vi "HAPS_MCU_Preamp_CMD.vi"(5 "set_Preamp":T3={"ch"=0, "chain_id"=0, "group"=3, "array_id"=0, "ele_phase"=0, "ele_gain"=0, "com_gain"=0, "pd_range"=0}, 7 "HAPS_MCU_Preamp_Func.":T2(ring), 8 "error in":errorcluster, 11 "Function":T1={"Tx/Rx"=enum."Rx", "Enable?"=enum."On", "Source"=enum."MCU"}) -> (0 "error out":errorcluster, 3 "Data":string)   [LabVIEW 2023, in "HAPS.lvlib"]
uses:
  HAPS.lvlib
  set_Preamp.ctl
  MCU_Function.ctl
panel:
  out "Time(ms)":dbl
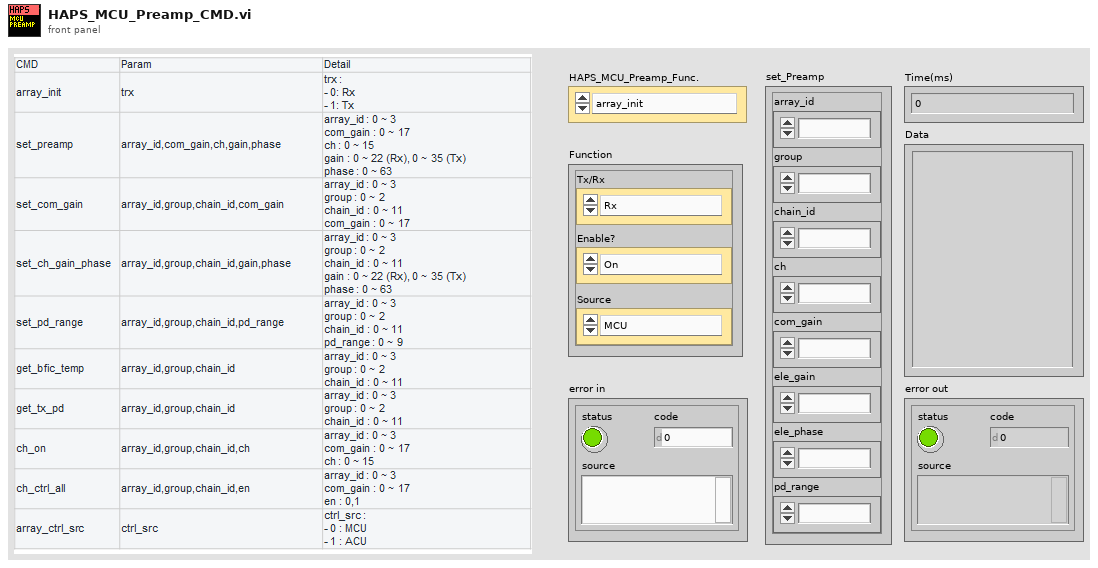
[diagram p1: front panel]
types:
  T1 = typedef "HAPS.lvlib/MCU_Function.ctl" = cluster{"Tx/Rx":enum16{"Rx", "Tx"}, "Enable?":enum16{"OFF", "On"}, "Source":enum16{"MCU", "ACU"}}
  T2 = enum16{"array_init", "set_preamp", "set_com_gain", "set_ch_gain_phase", "set_pd_range", "get_bfic_temp", "get_tx_pd", "ch_on", "ch_ctrl_all", "array_ctrl_src"}
  T3 = typedef "HAPS.lvlib/set_Preamp.ctl" = cluster{"ch":i32, "chain_id":i32, "group":i32, "array_id":i32, "ele_phase":i32, "ele_gain":i32, "com_gain":i32, "pd_range":i32}
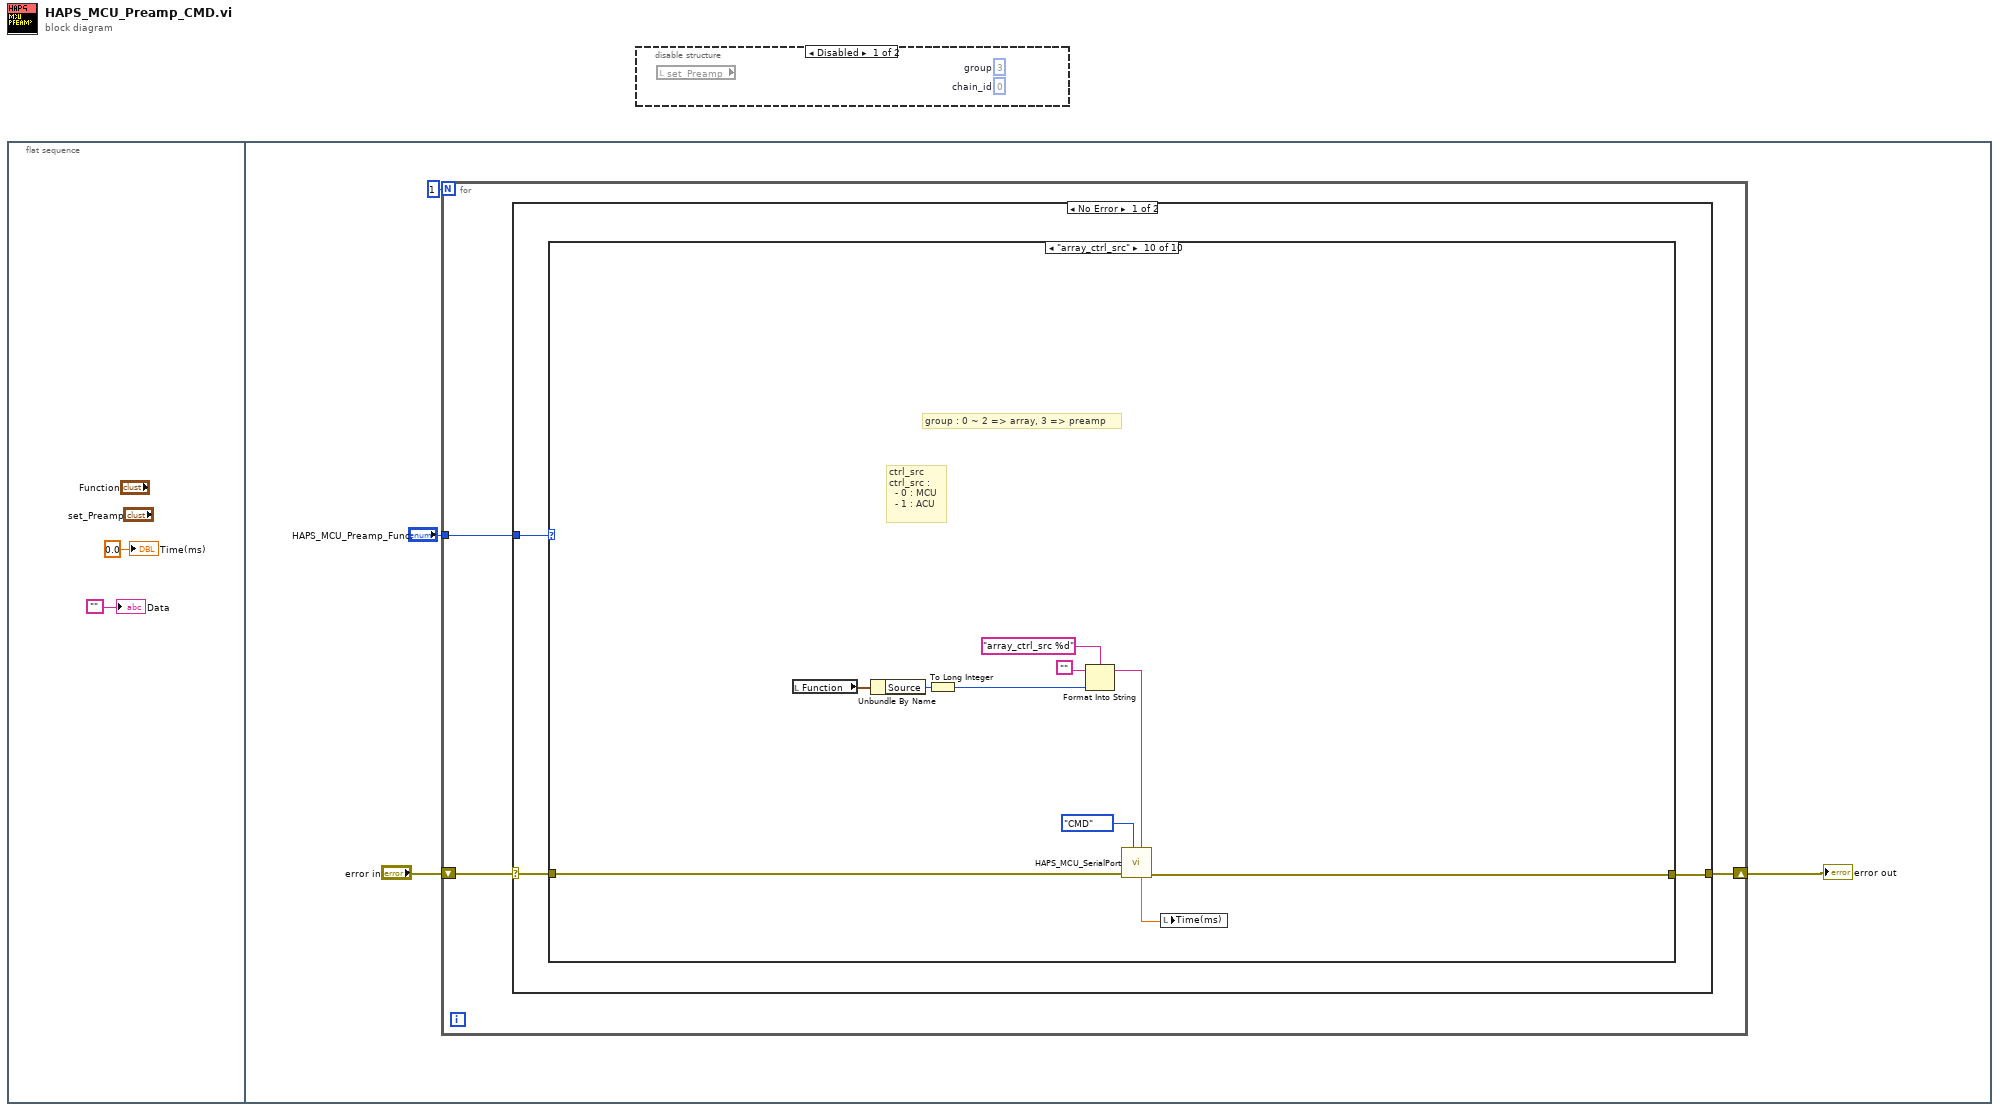
[diagram p0: block diagram]
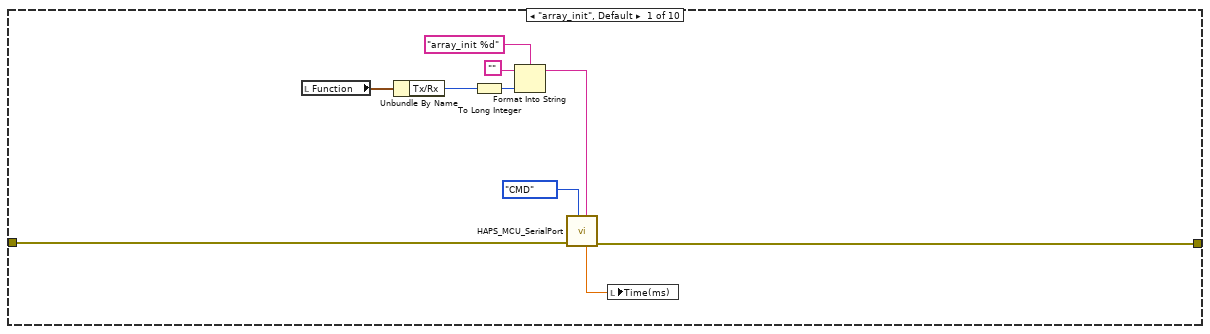
[diagram p3: hidden frame]
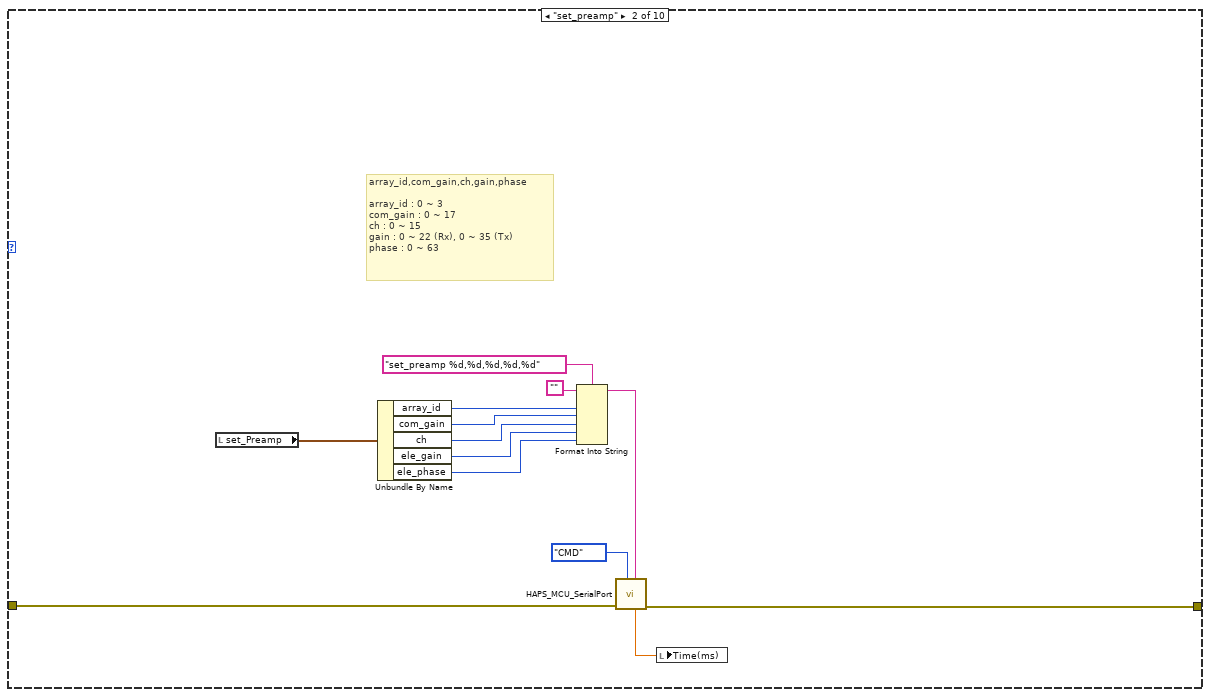
[diagram p4: hidden frame]
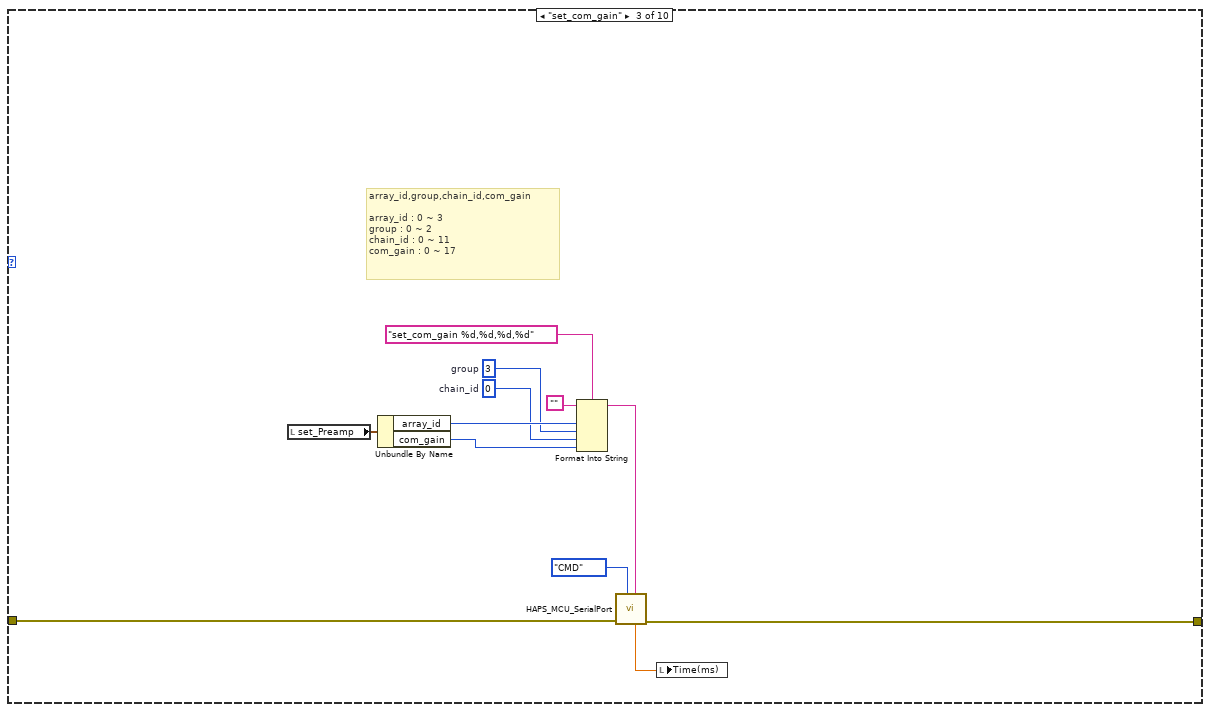
[diagram p5: hidden frame]
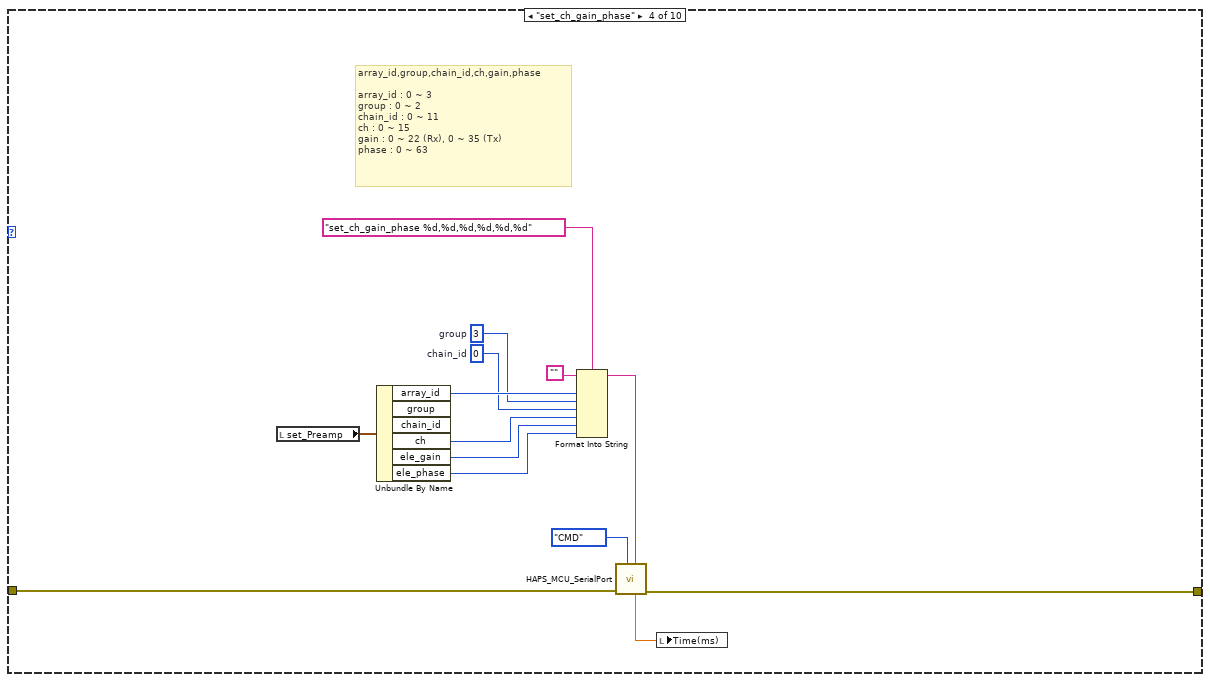
[diagram p6: hidden frame]
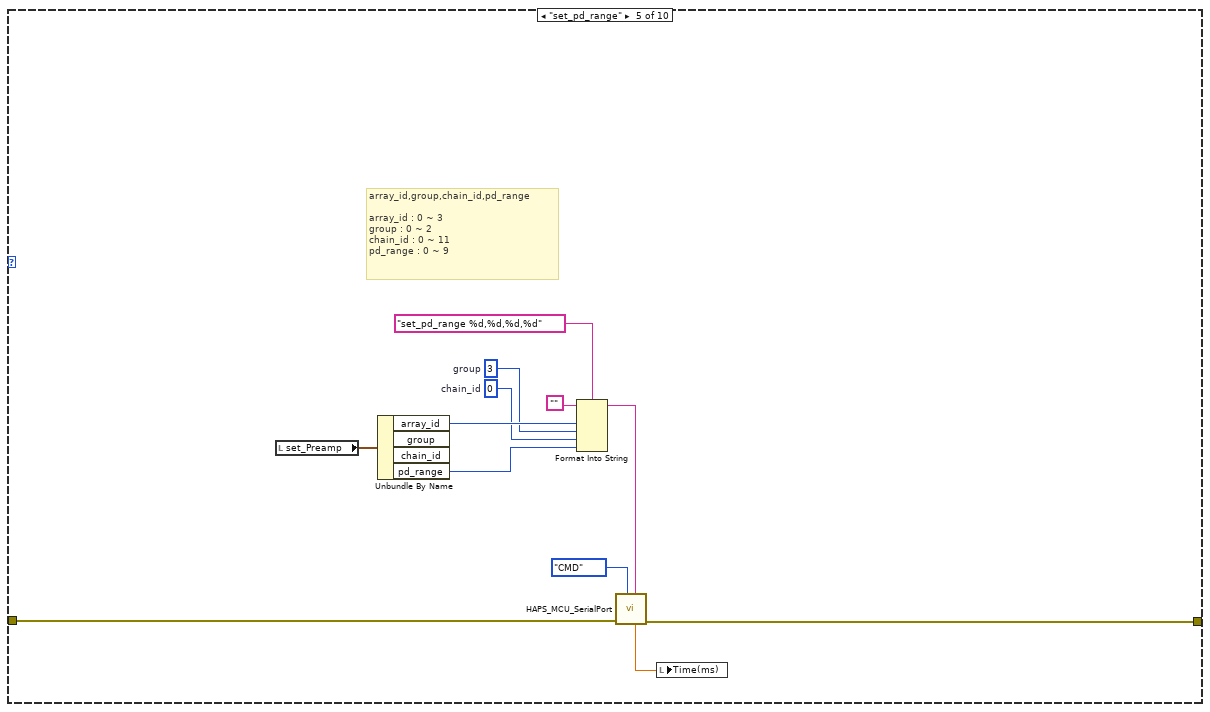
[diagram p7: hidden frame]
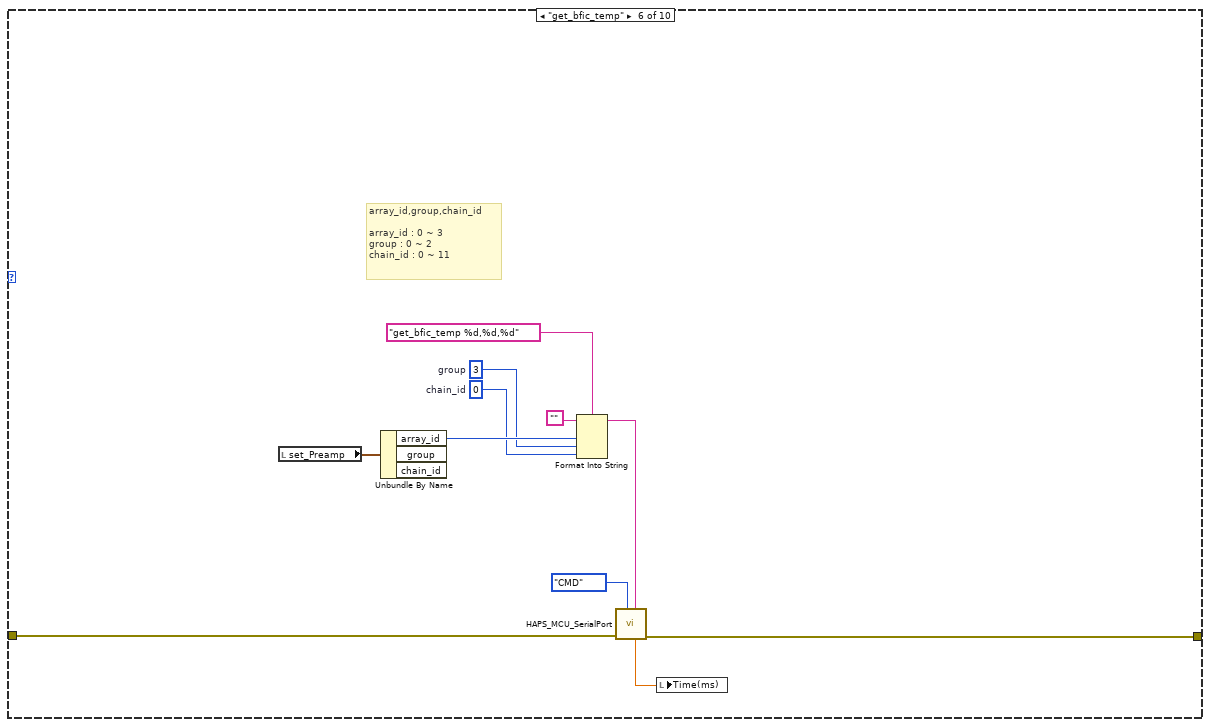
[diagram p8: hidden frame]
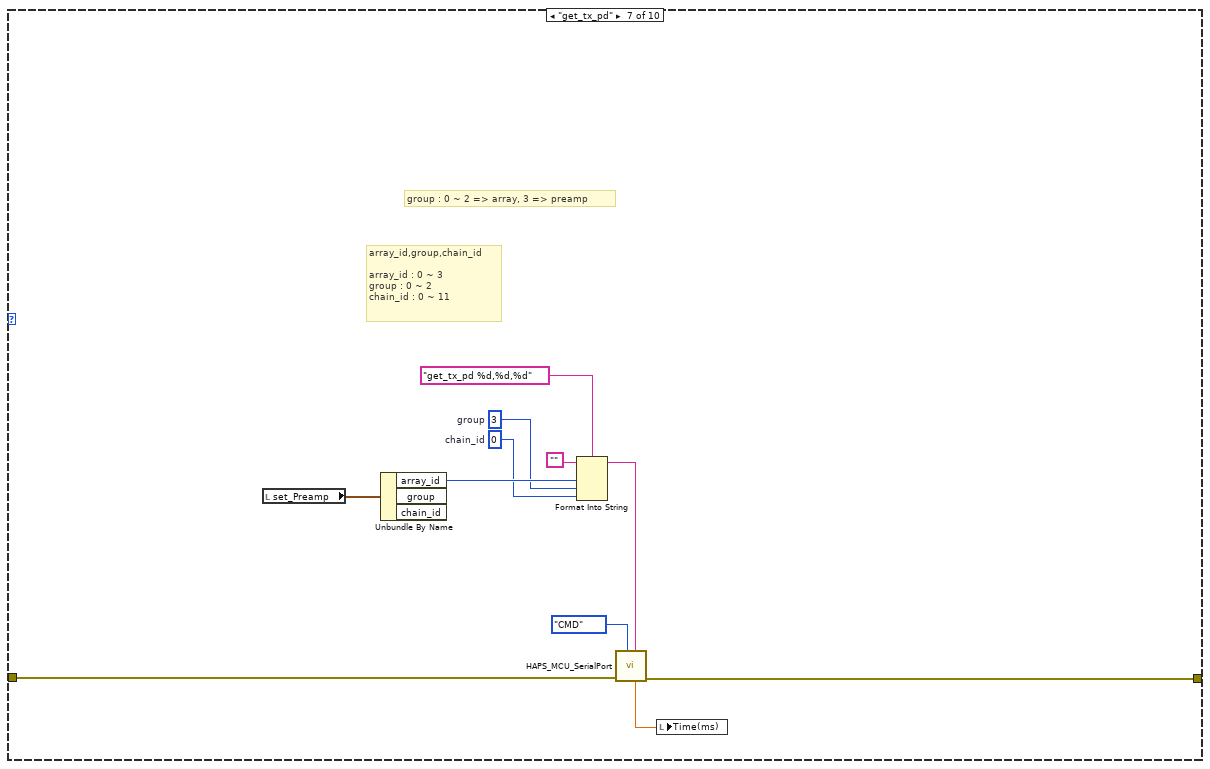
[diagram p9: hidden frame]
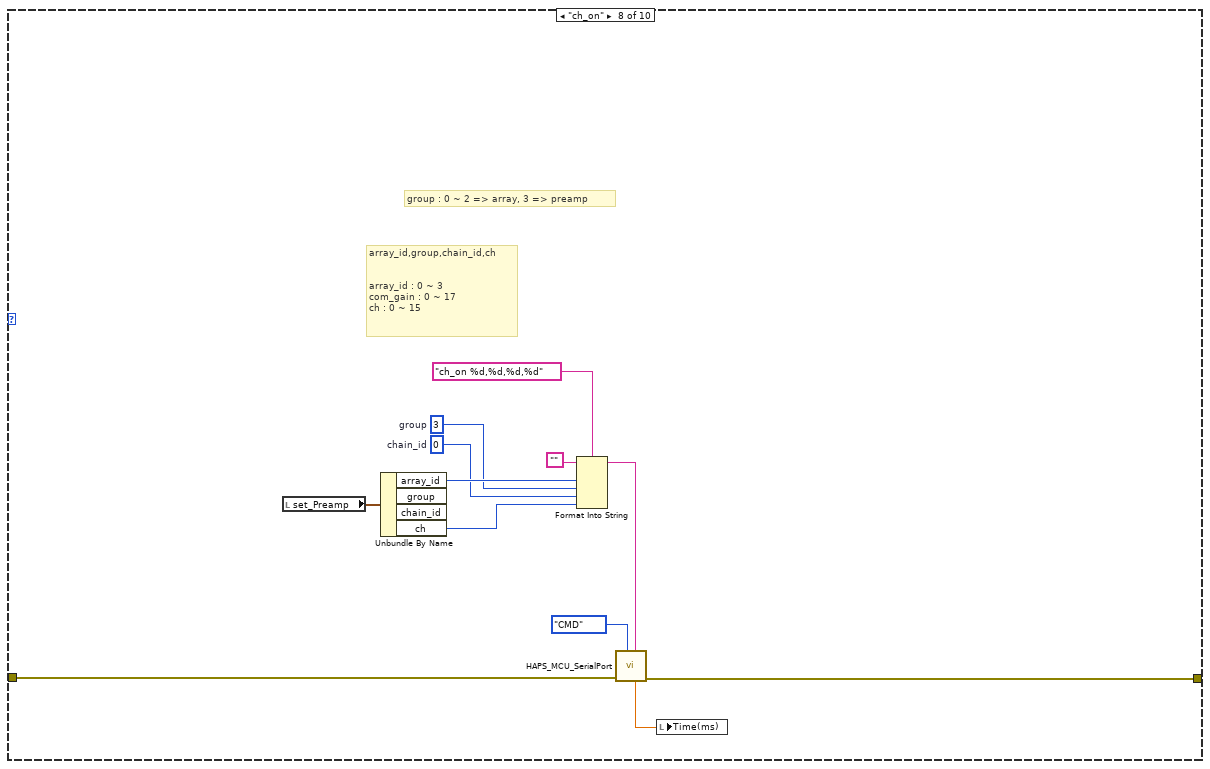
[diagram p10: hidden frame]
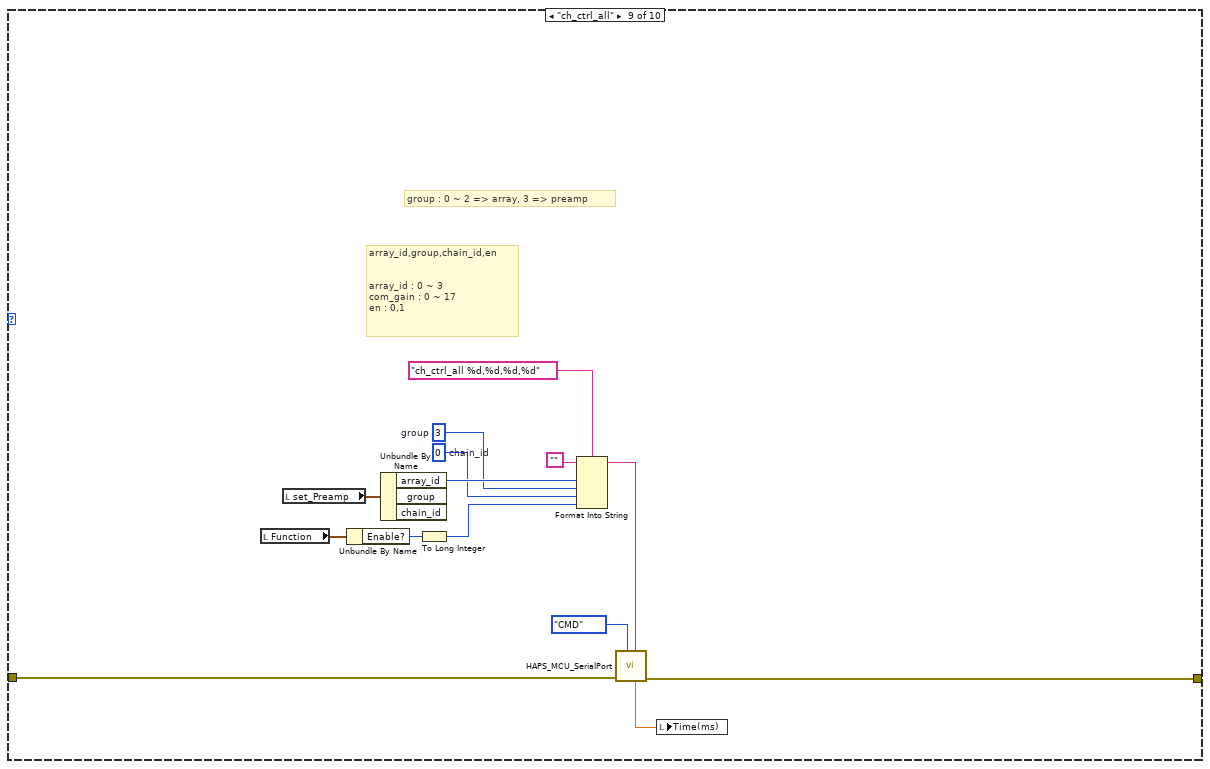
[diagram p11: hidden frame]
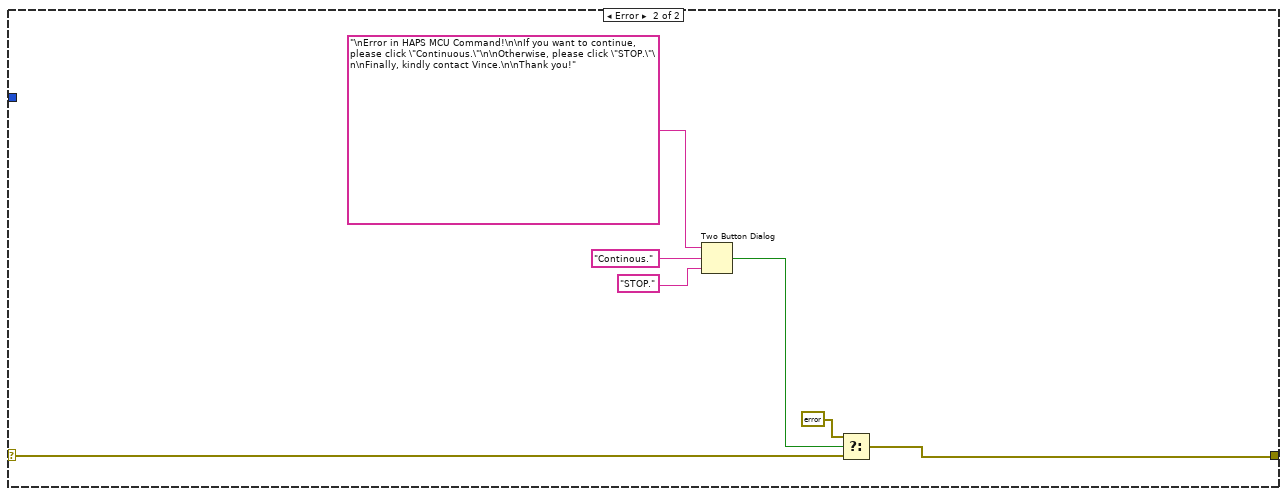
[diagram p12: hidden frame]
diagram:
  n1 = flat-sequence {
    frame #0 {
      "Time(ms)" <- 0.0 ("Time(ms)")
      "Data" <- ""
    }
    frame #1 {
      n2 = for {
        N: 1 -> [_]
        tunnel: "HAPS_MCU_Preamp_Func." -> [w7]
        shift-right: [w9] -> w3
        shift-left: "error in" -> [w8]
        n3 = case shown="No Error" w8 {
          selector: w8 -> [w12 w134]
          tunnel: [w10 w132] -> w9
          tunnel: w7 -> [w11 _]
          frame No Error {
            n4 = case shown="\"array_ctrl_src\"" w11 {
              tunnel: w12 -> [w22 w35 w47 w61 w73 w84 w95 w107 w121 w131]
              tunnel: [w21 w34 w46 w60 w72 w83 w94 w106 w120 w130] -> w10
              frame "array_init", Default {
                n5 = local read "Function"() -> (w16:T1)
                n6 = Unbundle By Name(w16) -> ("Tx/Rx"=w13:enum16{"Rx", "Tx"})
                n7 = To Long Integer(number=w13) -> (32bit integer=w15:i32)
                n8 = Format Into String(format string="array_init %d" ("Command"), initial string="", w15) -> (resulting string=w14:string)  [unwired: 1 in, 1 out]
                n9 = call "HAPS_MCU_SerialPort.vi"("Command"=w14, "HAPS_SerialPort_Func"=enum16{"Init", "Close", "CMD"}."CMD" ("HAPS_SerialPort"), "error in"=w22) -> ("error out"=w21:errorcluster, "Time(ms)"=w20:dbl)  [unwired: 6 in, 1 out]
                n10 = local write "Time(ms)"(w20) -> ()
              }
              frame "set_preamp" {
                # "array_id,com_gain,ch,gain,phase\n\narray_id : 0 ~ 3\ncom_gain : 0 ~ 17\nch : 0 ~ 15\ngain : 0 ~ 22 (Rx), 0 ~ 35 (Tx)\nphase : 0 ~ 63"
                n11 = local read "set_Preamp"() -> (w23:T3)
                n12 = Unbundle By Name(w23) -> ("array_id"=w28:i32, "com_gain"=w27:i32, "ch"=w26:i32, "ele_gain"=w25:i32, "ele_phase"=w24:i32)
                n13 = Format Into String(format string="set_preamp %d,%d,%d,%d,%d" ("Command"), initial string="", w28, w27, w26, w25, w24) -> (resulting string=w29:string)  [unwired: 1 in, 1 out]
                n14 = call "HAPS_MCU_SerialPort.vi"("Command"=w29, "HAPS_SerialPort_Func"=enum16{"Init", "Close", "CMD"}."CMD" ("HAPS_SerialPort"), "error in"=w35) -> ("error out"=w34:errorcluster, "Time(ms)"=w33:dbl)  [unwired: 6 in, 1 out]
                n15 = local write "Time(ms)"(w33) -> ()
              }
              frame "set_com_gain" {
                w37 = 0  # chain_id
                w38 = 3  # group
                # "array_id,group,chain_id,com_gain\n\narray_id : 0 ~ 3\ngroup : 0 ~ 2\nchain_id : 0 ~ 11\ncom_gain : 0 ~ 17"
                n16 = local read "set_Preamp"() -> (w39:T3)
                n17 = Unbundle By Name(w39) -> ("array_id"=w40:i32, "com_gain"=w36:i32)
                n18 = Format Into String(format string="set_com_gain %d,%d,%d,%d" ("Command"), initial string="", w40, w38, w37, w36) -> (resulting string=w41:string)  [unwired: 1 in, 1 out]
                n19 = call "HAPS_MCU_SerialPort.vi"("Command"=w41, "HAPS_SerialPort_Func"=enum16{"Init", "Close", "CMD"}."CMD" ("HAPS_SerialPort"), "error in"=w47) -> ("error out"=w46:errorcluster, "Time(ms)"=w45:dbl)  [unwired: 6 in, 1 out]
                n20 = local write "Time(ms)"(w45) -> ()
              }
              frame "set_ch_gain_phase" {
                w48 = 0  # chain_id
                w49 = 3  # group
                # "array_id,group,chain_id,ch,gain,phase\n\narray_id : 0 ~ 3\ngroup : 0 ~ 2\nchain_id : 0 ~ 11\nch : 0 ~ 15\ngain : 0 ~ 22 (Rx), 0 ~ 35 (Tx)\nphase : 0 ~ 63"
                n21 = local read "set_Preamp"() -> (w52:T3)
                n22 = Unbundle By Name(w52) -> ("array_id"=w54:i32, "ch"=w53:i32, "ele_gain"=w51:i32, "ele_phase"=w50:i32)  [unwired: 2 out]
                n23 = Format Into String(format string="set_ch_gain_phase %d,%d,%d,%d,%d,%d" ("Command"), initial string="", w54, w49, w48, w53, w51, w50) -> (resulting string=w55:string)  [unwired: 1 in, 1 out]
                n24 = call "HAPS_MCU_SerialPort.vi"("Command"=w55, "HAPS_SerialPort_Func"=enum16{"Init", "Close", "CMD"}."CMD" ("HAPS_SerialPort"), "error in"=w61) -> ("error out"=w60:errorcluster, "Time(ms)"=w59:dbl)  [unwired: 6 in, 1 out]
                n25 = local write "Time(ms)"(w59) -> ()
              }
              frame "set_pd_range" {
                w63 = 0  # chain_id
                w62 = 3  # group
                # "array_id,group,chain_id,pd_range\n\narray_id : 0 ~ 3\ngroup : 0 ~ 2\nchain_id : 0 ~ 11\npd_range : 0 ~ 9"
                n26 = local read "set_Preamp"() -> (w64:T3)
                n27 = Unbundle By Name(w64) -> ("array_id"=w66:i32, "pd_range"=w65:i32)  [unwired: 2 out]
                n28 = Format Into String(format string="set_pd_range %d,%d,%d,%d" ("Command"), initial string="", w66, w62, w63, w65) -> (resulting string=w67:string)  [unwired: 1 in, 1 out]
                n29 = call "HAPS_MCU_SerialPort.vi"("Command"=w67, "HAPS_SerialPort_Func"=enum16{"Init", "Close", "CMD"}."CMD" ("HAPS_SerialPort"), "error in"=w73) -> ("error out"=w72:errorcluster, "Time(ms)"=w71:dbl)  [unwired: 6 in, 1 out]
                n30 = local write "Time(ms)"(w71) -> ()
              }
              frame "get_bfic_temp" {
                w75 = 0  # chain_id
                w74 = 3  # group
                # "array_id,group,chain_id\n\narray_id : 0 ~ 3\ngroup : 0 ~ 2\nchain_id : 0 ~ 11"
                n31 = local read "set_Preamp"() -> (w76:T3)
                n32 = Unbundle By Name(w76) -> ("array_id"=w77:i32)  [unwired: 2 out]
                n33 = Format Into String(format string="get_bfic_temp %d,%d,%d" ("Command"), initial string="", w77, w74, w75) -> (resulting string=w78:string)  [unwired: 1 in, 1 out]
                n34 = call "HAPS_MCU_SerialPort.vi"("Command"=w78, "HAPS_SerialPort_Func"=enum16{"Init", "Close", "CMD"}."CMD" ("HAPS_SerialPort"), "error in"=w84) -> ("error out"=w83:errorcluster, "Time(ms)"=w82:dbl)  [unwired: 6 in, 1 out]
                n35 = local write "Time(ms)"(w82) -> ()
              }
              frame "get_tx_pd" {
                w86 = 0  # chain_id
                w85 = 3  # group
                # "group : 0 ~ 2 => array, 3 => preamp"
                # "array_id,group,chain_id\n\narray_id : 0 ~ 3\ngroup : 0 ~ 2\nchain_id : 0 ~ 11"
                n36 = local read "set_Preamp"() -> (w87:T3)
                n37 = Unbundle By Name(w87) -> ("array_id"=w88:i32)  [unwired: 2 out]
                n38 = Format Into String(format string="get_tx_pd %d,%d,%d" ("Command"), initial string="", w88, w85, w86) -> (resulting string=w89:string)  [unwired: 1 in, 1 out]
                n39 = call "HAPS_MCU_SerialPort.vi"("Command"=w89, "HAPS_SerialPort_Func"=enum16{"Init", "Close", "CMD"}."CMD" ("HAPS_SerialPort"), "error in"=w95) -> ("error out"=w94:errorcluster, "Time(ms)"=w93:dbl)  [unwired: 6 in, 1 out]
                n40 = local write "Time(ms)"(w93) -> ()
              }
              frame "ch_on" {
                w97 = 0  # chain_id
                w96 = 3  # group
                # "group : 0 ~ 2 => array, 3 => preamp"
                # "array_id,group,chain_id,ch\n\n\narray_id : 0 ~ 3\ncom_gain : 0 ~ 17\nch : 0 ~ 15"
                n41 = local read "set_Preamp"() -> (w99:T3)
                n42 = Unbundle By Name(w99) -> ("array_id"=w100:i32, "ch"=w98:i32)  [unwired: 2 out]
                n43 = Format Into String(format string="ch_on %d,%d,%d,%d" ("Command"), initial string="", w100, w96, w97, w98) -> (resulting string=w101:string)  [unwired: 1 in, 1 out]
                n44 = call "HAPS_MCU_SerialPort.vi"("Command"=w101, "HAPS_SerialPort_Func"=enum16{"Init", "Close", "CMD"}."CMD" ("HAPS_SerialPort"), "error in"=w107) -> ("error out"=w106:errorcluster, "Time(ms)"=w105:dbl)  [unwired: 6 in, 1 out]
                n45 = local write "Time(ms)"(w105) -> ()
              }
              frame "ch_ctrl_all" {
                w110 = 0  # chain_id
                w109 = 3  # group
                # "group : 0 ~ 2 => array, 3 => preamp"
                # "array_id,group,chain_id,en\n\n\narray_id : 0 ~ 3\ncom_gain : 0 ~ 17\nen : 0,1"
                n46 = local read "Function"() -> (w112:T1)
                n47 = local read "set_Preamp"() -> (w113:T3)
                n48 = Unbundle By Name(w112) -> ("Enable?"=w108:enum16{"OFF", "On"})
                n49 = Unbundle By Name(w113) -> ("array_id"=w114:i32)  [unwired: 2 out]
                n50 = To Long Integer(number=w108) -> (32bit integer=w111:i32)
                n51 = Format Into String(format string="ch_ctrl_all %d,%d,%d,%d" ("Command"), initial string="", w114, w109, w110, w111) -> (resulting string=w115:string)  [unwired: 1 in, 1 out]
                n52 = call "HAPS_MCU_SerialPort.vi"("Command"=w115, "HAPS_SerialPort_Func"=enum16{"Init", "Close", "CMD"}."CMD" ("HAPS_SerialPort"), "error in"=w121) -> ("error out"=w120:errorcluster, "Time(ms)"=w119:dbl)  [unwired: 6 in, 1 out]
                n53 = local write "Time(ms)"(w119) -> ()
              }
              frame "array_ctrl_src" {
                # "group : 0 ~ 2 => array, 3 => preamp"
                # "ctrl_src\nctrl_src : \n  - 0 : MCU\n  - 1 : ACU"
                n54 = local read "Function"() -> (w124:T1)
                n55 = Unbundle By Name(w124) -> ("Source"=w122:enum16{"MCU", "ACU"})
                n56 = To Long Integer(number=w122) -> (32bit integer=w123:i32)
                n57 = Format Into String(format string="array_ctrl_src %d" ("Command"), initial string="", w123) -> (resulting string=w125:string)  [unwired: 1 in, 1 out]
                n58 = call "HAPS_MCU_SerialPort.vi"("Command"=w125, "HAPS_SerialPort_Func"=enum16{"Init", "Close", "CMD"}."CMD" ("HAPS_SerialPort"), "error in"=w131) -> ("error out"=w130:errorcluster, "Time(ms)"=w129:dbl)  [unwired: 6 in, 1 out]
                n59 = local write "Time(ms)"(w129) -> ()
              }
            }
          }
          frame Error {
            n60 = Two Button Dialog(message="\nError in HAPS MCU Command!\n\nIf you want to continue, please click \"Continuous.\"\n\nOtherwise, please click \"STOP.\"\n\nFinally, kindly contact Vince.\n\nThank you!", 1:"STOP." ("F button name (\"Cancel\")"), 2:"Continous." ("T button name (\"OK\")")) -> (T button?=w135:bool)
            n61 = Select(t=errorcluster {"status"=FALSE, "code"=0, "source"=""}, s=w135, f=w134) -> (s? t:f=w132:errorcluster)
          }
        }
      }
      "error out" <- w3
    }
  }
  n62 = disable-structure shown="Disabled" {
    frame Disabled {
      (unwired) 0  # chain_id
      (unwired) 3  # group
      n63 = local read "set_Preamp"() -> ()  [unwired: 1 out]
    }
    frame Enabled {
    }
  }
